vi "SavedSettingsTitleAndDescription.vi"(8 "error in (no error)":errorcluster, 10 "Tag":string, 11 "TreeControl in":refnum<vi>) -> (0 "error out":errorcluster, 1 "Description":string="(Add comment for this setting.)", 2 "Title":string="New Setting", 3 "reference out":refnum<vi>, 4 "Value":string)   [LabVIEW 2019]
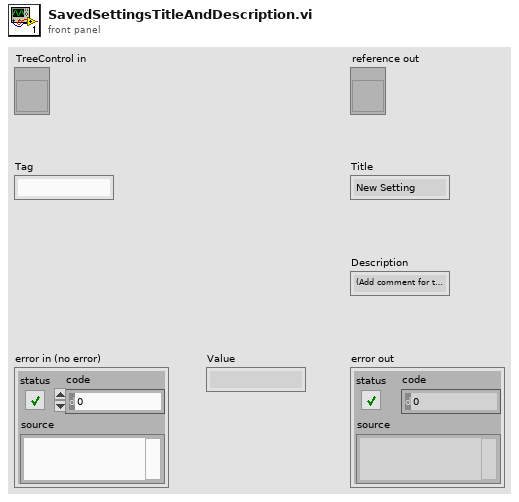
[diagram p1: front panel]
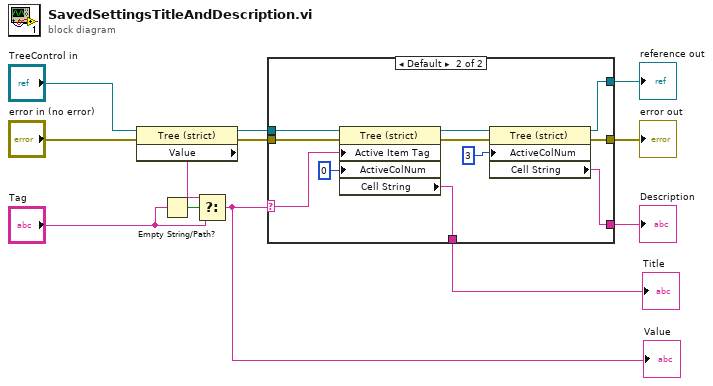
[diagram p0: block diagram]
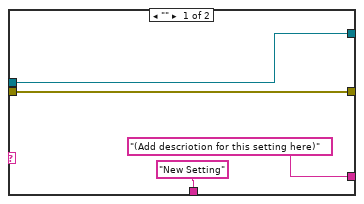
[diagram p2: hidden frame]
diagram:
  n1 = property class="Tree (strict)"(reference="TreeControl in", error in="error in (no error)") -> (reference out=w9:refnum<vi>, error out=w7:errorcluster, "Value"=w4:string)
  n2 = Empty String/Path?(string/path="Tag") -> (empty?=w2:bool)
  n3 = Select(t=w4, s=w2, f="Tag") -> (s? t:f=w1:string)
  "Value" <- w1
  n4 = case shown="Default" w1 {
    selector: w1 -> [_ w17]
    tunnel: ["New Setting" ("Cell String") w24] -> w11
    tunnel: ["(Add descriotion for this setting here)" ("Cell String") w23] -> w10
    tunnel: w9 -> [w13 w22]
    tunnel: [w13 w21] -> w8
    tunnel: w7 -> [w14 w20]
    tunnel: [w14 w18] -> w6
    frame "" {
    }
    frame Default {
      n5 = property class="Tree (strict)"(reference=w22, error in=w20, "Active Item Tag"=w17, "ActiveColNum"=0 ("Active Cell:Active Column Number")) -> (reference out=w27:refnum<vi>, error out=w19:errorcluster, "Cell String"=w24:string)
      n6 = property class="Tree (strict)"(reference=w27, error in=w19, "ActiveColNum"=3 ("Active Cell:Active Column Number")) -> (reference out=w21:refnum<vi>, error out=w18:errorcluster, "Cell String"=w23:string)
    }
  }
  "Title" <- w11
  "Description" <- w10
  "error out" <- w6
  "reference out" <- w8
